vi "PopulateColorMode.vi"(9 "Bayer pattern":refnum<vi>, 10 "ColorMode":refnum<k24>, 11 "String in":refnum<vi>) -> ()   [LabVIEW 2018]
uses:
  D:/SVN/PM/sdk/AppSamples/LabVIEWSamples/trunk/Release/2018/Dependencies/PVCamNET.dll
  Dependencies/PVCamNET.dll
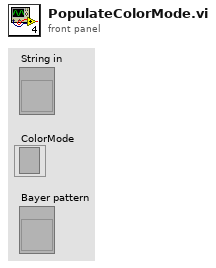
[diagram p1: front panel]
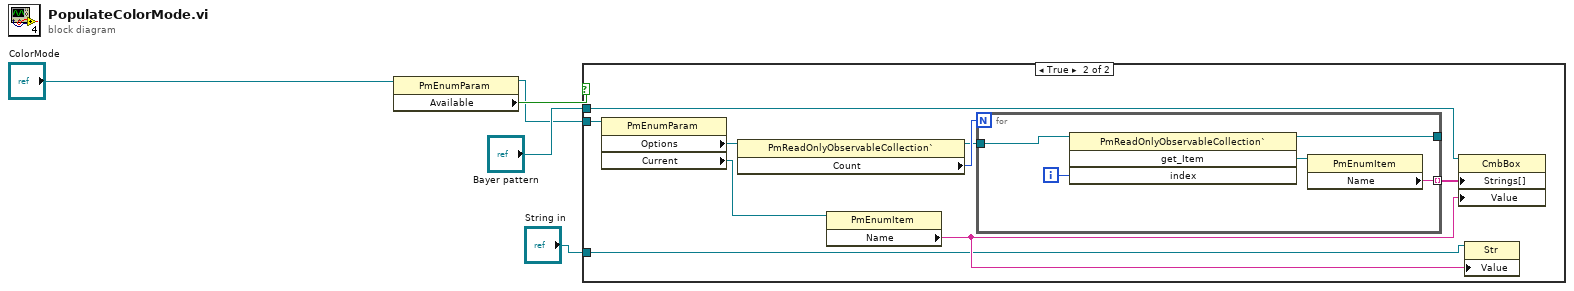
[diagram p0: block diagram]
diagram:
  n1 = property class="PmEnumParam"(reference="ColorMode") -> (reference out=w2:refnum<k24>, "Available"=w3:bool)  [unwired: 1 in, 1 out]
  n2 = case shown="True" w3 {
    tunnel: "Bayer pattern" -> [_ w13]
    tunnel: w2 -> [_ w12]
    tunnel: "String in" -> [_ w6]
    frame False {
    }
    frame True {
      n3 = property class="PmEnumParam"(reference=w12) -> ("Options"=w11:refnum<k24>, "Current"=w8:refnum<k24>)  [unwired: 1 in, 2 out]
      n4 = property class="PmReadOnlyObservableCollection`"(reference=w11) -> (reference out=w9:refnum<k24>, "Count"=w10:i32)  [unwired: 1 in, 1 out]
      n5 = property class="PmEnumItem"(reference=w8) -> ("Name"=w7:string)  [unwired: 1 in, 2 out]
      n6 = for {
        N: w10 -> [_]
        tunnel: [w19] -> w14 mode=indexing
        tunnel: [w15] -> _
        tunnel: w9 -> [w18]
        i -> [w17]
        n7 = invoke class="PmReadOnlyObservableCollection`" method="get_Item"(reference=w18, "index"=w17) -> (reference out=w15:refnum<k24>, "get_Item"=w16:refnum<k24>)  [unwired: 2 in, 2 out]
        n8 = property class="PmEnumItem"(reference=w16) -> ("Name"=w19:string)  [unwired: 1 in, 2 out]
      }
      n9 = property class="CmbBox"(reference=w13, "Strings[]"=w14, "Value"=w7) -> ()  [unwired: 1 in, 2 out]
      n10 = property class="Str"(reference=w6, "Value"=w7) -> ()  [unwired: 1 in, 2 out]
    }
  }
